vi "Write ADU Packet.vi"(8 "error in (no error)":errorcluster, 9 "modbus data unit":refnum<class "Modbus Data Unit (PDU).lvclass">, 10 "protocol layer":refnum<class "Network Protocol.lvclass">, 11 "IP transmission data unit in":refnum<class "IP Data Unit.lvclass">) -> (0 "error out":errorcluster, 2 "protocol layer out":refnum<class "Network Protocol.lvclass">, 3 "IP transmission data unit out":refnum<class "IP Data Unit.lvclass">)   [LabVIEW 2020, in "SubVIs.lvlib" / "IP Data Unit.lvclass"]
doc: "This uses the protocol layer to write a modbus packet to the bus, wrapped in the IP transmission data unit."
uses:
  <vilib>/Modbus/subvis/Transmission Data Unit (ADU)/IP Data Unit/IP Data Unit.lvclass
  C:/builds/penguin/iak/lvdsc/trunk/20.0/lv/vi.lib/Modbus/subvis/Transmission Data Unit (ADU)/Transmission Data Unit/Transmission Data Unit.lvclass
  <vilib>/Modbus/subvis/Modbus Data Unit (PDU)/Modbus Data Unit (PDU).lvclass
  <vilib>/Modbus/subvis/Protocol/Interfaces/Network Protocol/Network Protocol.lvclass
  <vilib>/Modbus/subvis/Transmission Data Unit (ADU)/Transmission Data Unit/Transmission Data Unit.lvclass/Transmission Data Unit.ctl
  <vilib>/Modbus/subvis/Transmission Data Unit (ADU)/IP Data Unit/IP Data Unit.lvclass/IP Data Unit.ctl
  <vilib>/Modbus/subvis/Modbus Data Unit (PDU)/Modbus Data Unit (PDU).lvclass/Modbus Data Unit (PDU).ctl
  <vilib>/Modbus/subvis/Transmission Data Unit (ADU)/Transmission Data Unit/Transmission Data Unit.lvclass
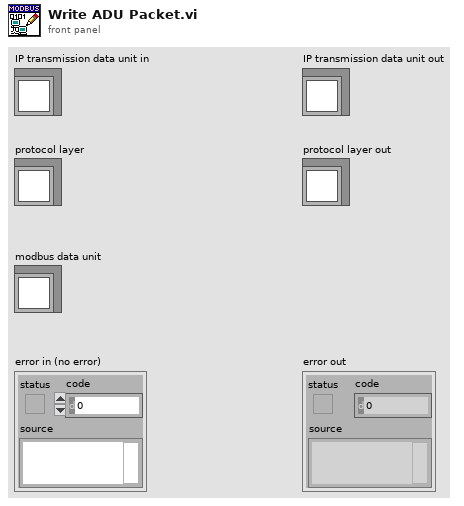
[diagram p1: front panel]
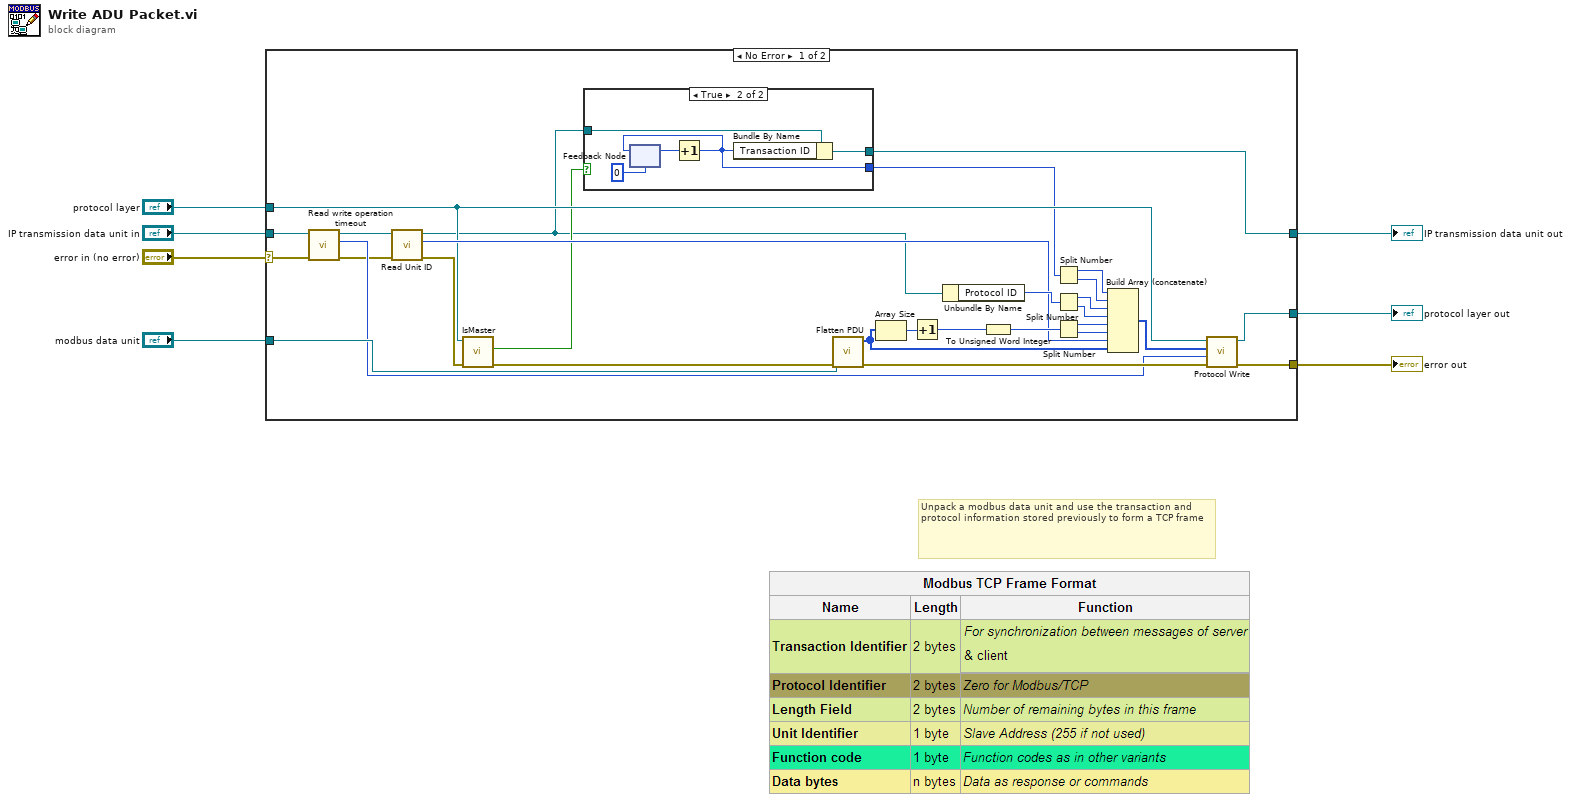
[diagram p0: block diagram]
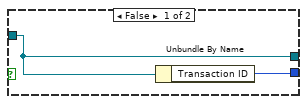
[diagram p2: hidden frame]
diagram:
  # "Unpack a modbus data unit and use the transaction and protocol information stored previously to form a TCP frame"
  n1 = case shown="No Error" "error in (no error)" {
    selector: "error in (no error)" -> [w15 w44]
    tunnel: [w36 w44] -> w7
    tunnel: "protocol layer" -> [w12 w45]
    tunnel: "modbus data unit" -> [w35 _]
    tunnel: [w34 w45] -> w4
    tunnel: "IP transmission data unit in" -> [w16 w46]
    tunnel: [w8 w46] -> w2
    frame No Error {
      n2 = call <vilib>:"Read write operation timeout.vi"("error in (no error)"=w15, "transmission data unit in"=w16) -> ("error out"=w18:errorcluster, "write operation timeout"=w19:i32, "transmission data unit out"=w17:refnum<class "IP Data Unit.lvclass">)  [unwired: 7 in]
      n3 = call <vilib>:"Read Unit ID.vi"("error in"=w18, "transmission data unit in"=w17) -> ("error out"=w14:errorcluster, "unit ID"=w20:u8, "transmission data unit out"=w10:refnum<class "IP Data Unit.lvclass">)  [unwired: 7 in]
      n4 = call-dynamic "IsMaster.vi"("error in (no error)"=w14, "Network Protocol in"=w12) -> ("error out"=w13:errorcluster, "isMaster"=w11:bool)  [unwired: 7 in, 1 out]
      n5 = case shown="True" w11 {
        tunnel: w10 -> [w37 w42]
        tunnel: [w37 w40] -> w8
        tunnel: [w38 w39] -> w9
        frame False {
          n6 = Unbundle By Name(w37) -> ("Transaction ID"=w38:u16)
        }
        frame True {
          n7 = feedback #1(u16 0) -> (w41:u16)
          n8 = Increment(x=w41) -> (x+1=w39:u16)
          n9 = feedback-in #1(w39) -> ()
          n10 = Bundle By Name(cluster=w42, "Transaction ID"=w39) -> (w40:refnum<class "IP Data Unit.lvclass">)
        }
      }
      n11 = call <vilib>:"Flatten PDU.vi"("error in (no error)"=w13, "Modbus data unit in"=w35) -> ("error out"=w22:errorcluster, "full Modbus data unit"=w21:u8[])  [unwired: 8 in]
      n12 = Array Size(array=w21) -> (size(s)=w33:i32)
      n13 = Increment(x=w33) -> (x+1=w31:i32)
      n14 = Unbundle By Name(w10) -> ("Protocol ID"=w32:u16)
      n15 = To Unsigned Word Integer(number=w31) -> (unsigned 16bit integer=w30:u16)
      n16 = Split Number(x=w9) -> (hi(x)=w29:u8, lo(x)=w28:u8)
      n17 = Split Number(x=w32) -> (hi(x)=w27:u8, lo(x)=w26:u8)
      n18 = Split Number(x=w30) -> (hi(x)=w25:u8, lo(x)=w24:u8)
      n19 = Build Array (concatenate)(w29, w28, w27, w26, w25, w24, w20, w21) -> (w23:u8[])
      n20 = call-dynamic "Protocol Write.vi"("error in (no error)"=w22, "timeout"=w19, "data"=w23, "protocol layer in"=w12) -> ("error out"=w36:errorcluster, "protocol layer out"=w34:refnum<class "Network Protocol.lvclass">)  [unwired: 5 in, 1 out]
    }
    frame Error {
    }
  }
  "error out" <- w7
  "IP transmission data unit out" <- w2
  "protocol layer out" <- w4
